vi "Get Metrics.vi"(7 "LabVIEW Web Service Request":refnum<class "Web Request.lvclass">, 11 "Registry":string="_default_registry") -> ()   [LabVIEW 2020]
uses:
  <vilib>/wsapi/Web Request.lvclass
  registry/session/Registry Session.lvclass
  metrics/metric/Metric.lvclass
panel:
  # "Use the Web Service Request input terminal to call the VIs on the Web Services palette. Do not remove it from the connector pane unless you don't need access to the palette."
  # "Each additional control wired to the connector pane will be available as an input in the URL. To include an indicator in terminal-mode output (the default setting), it must also be wired to the connector pane."
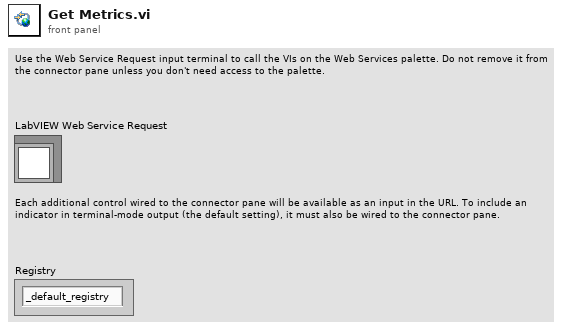
[diagram p1: front panel]
types:
  T1 = typedef "Registry.lvlib/Registry Session.lvclass/Session Handle.ctl" = refnum<data-value>
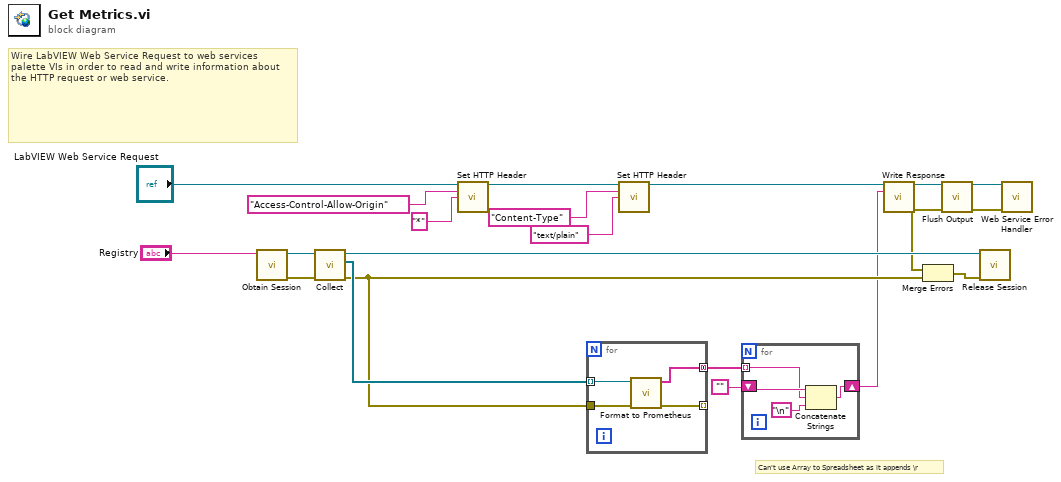
[diagram p0: block diagram]
diagram:
  # "Can't use Array to Spreadsheet as it appends \\r"
  # "Wire LabVIEW Web Service Request to web services palette VIs in order to read and write information about the HTTP request or web service."
  n1 = call "Obtain Session.vi"("Session  Name ()"="Registry") -> ("error out"=w16:errorcluster, "Session Handle"=w17:T1)  [unwired: 9 in]
  n2 = call "Collect.vi"("error in (no error)"=w16, "Session Handle in"=w17) -> ("error out"=w4:errorcluster, "Metrics"=w15:refnum<data-value>[], "Session Handle out"=w14:T1)  [unwired: 7 in]
  n3 = call <vilib>:"Set HTTP Header.vi"("LabVIEW Web Service Request"="LabVIEW Web Service Request", "header"="Access-Control-Allow-Origin", "header value"="*") -> ("LabVIEW Web Service Request out"=w8:refnum<class "Web Request.lvclass">)  [unwired: 11 in, 1 out]
  n4 = for {
    tunnel: w15 -> [w25] mode=indexing
    tunnel: [w24] -> w1 mode=concatenating
    tunnel: w4 -> [w23]
    tunnel: [w22] -> _ mode=indexing
    n5 = call "Format to Prometheus.vi"("error in (no error)"=w23, "Data Value Reference in"=w25) -> ("error out"=w22:errorcluster, "Prometheus-formatted Metric"=w24:string[])  [unwired: 8 in]
  }
  n6 = call <vilib>:"Set HTTP Header.vi"("LabVIEW Web Service Request"=w8, "header"="Content-Type", "header value"="text/plain") -> ("LabVIEW Web Service Request out"=w7:refnum<class "Web Request.lvclass">)  [unwired: 11 in, 1 out]
  n7 = for {
    tunnel: w1 -> [w27] mode=indexing
    shift-right: [w26] -> w2
    shift-left: "" -> [w29]
    n8 = Concatenate Strings(w29, w27, "\n") -> (w26:string)
  }
  n9 = call <vilib>:"Write Response.vi"("LabVIEW Web Service Request"=w7, "response string"=w2) -> ("LabVIEW Web Service Request out"=w13:refnum<class "Web Request.lvclass">, "error out"=w5:errorcluster)  [unwired: 12 in]
  n10 = Merge Errors(w5, w4) -> (w6:errorcluster)
  n11 = call <vilib>:"Flush Output.vi"("LabVIEW Web Service Request"=w13, "error in (no error)"=w5) -> ("LabVIEW Web Service Request out"=w11:refnum<class "Web Request.lvclass">, "error out"=w12:errorcluster)  [unwired: 12 in]
  n12 = call "Release Session.vi"("error in (no error)"=w6, "Session Handle"=w14) -> ()  [unwired: 9 in, 1 out]
  n13 = call "Web Service Error Handler.vi"("LabVIEW Web Service Request"=w11, "error in (no error)"=w12) -> ()  [unwired: 12 in, 2 out]
